vi "TrueAndFalseBasedCaseStructure.vi"() -> ()   [LabVIEW 2019]
panel:
  in  "a":dbl
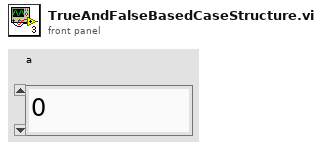
[diagram p1: front panel]
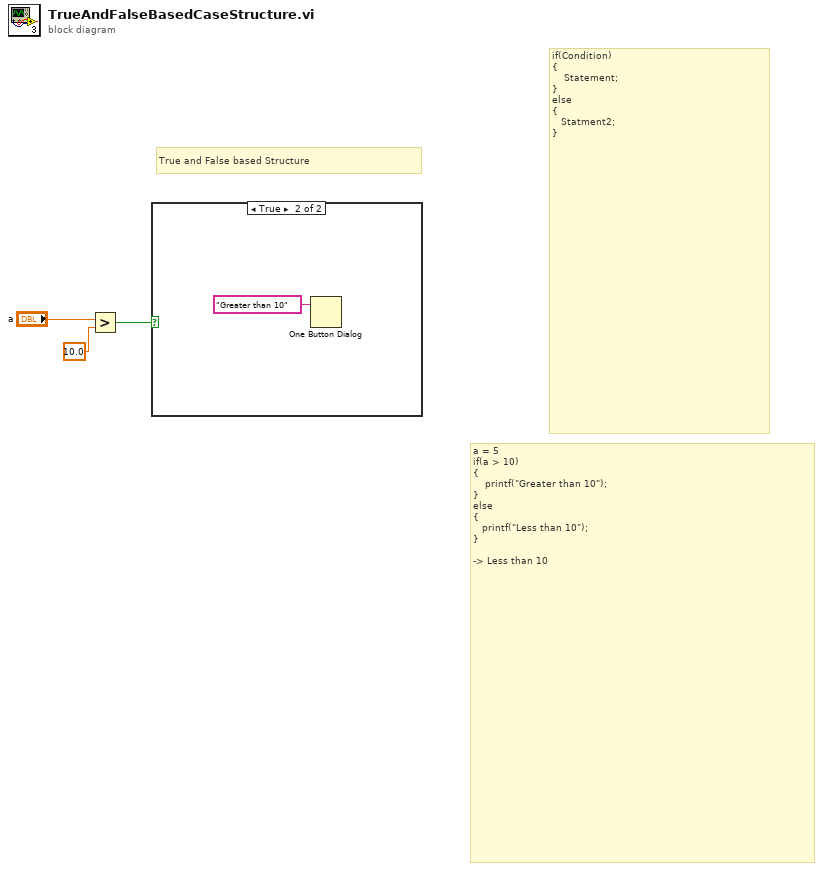
[diagram p0: block diagram]
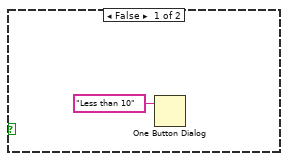
[diagram p2: hidden frame]
diagram:
  # "True and False based Structure"
  # "a = 5\nif(a > 10)\n{\n    printf(\"Greater than 10\");\n}\nelse\n{\n   printf(\"Less than 10\");\n}\n\n-> Less than 10"
  # "if(Condition)\n{\n    Statement;\n}\nelse\n{\n   Statment2;\n}"
  n1 = Greater?(x="a", y=10.0) -> (0:w1:bool)
  n2 = case shown="True" w1 {
    frame False {
      n3 = One Button Dialog(message="Less than 10") -> ()  [unwired: 1 in, 1 out]
    }
    frame True {
      n4 = One Button Dialog(message="Greater than 10") -> ()  [unwired: 1 in, 1 out]
    }
  }
